vi "Auto Get Server Message and Update UI.vi"(8 "error in (no error)":errorcluster, 10 "MQTT Data":T4, 11 "Data Cluster":T1) -> (0 "error out":errorcluster, 3 "Data Out":T1)   [LabVIEW 2017]
uses:
  controls/Auto UI Data.ctl
  controls/Configuration Details.ctl
  IPC/MQTT/Controls/Publish data.ctl
  <vilib>/vision/Image Controls.llb/IMAQ Image.ctl
  controls/Server CMDs to Publish.ctl
  Database/Controls/DB Options.ctl
panel:
  out "Image Out":T3
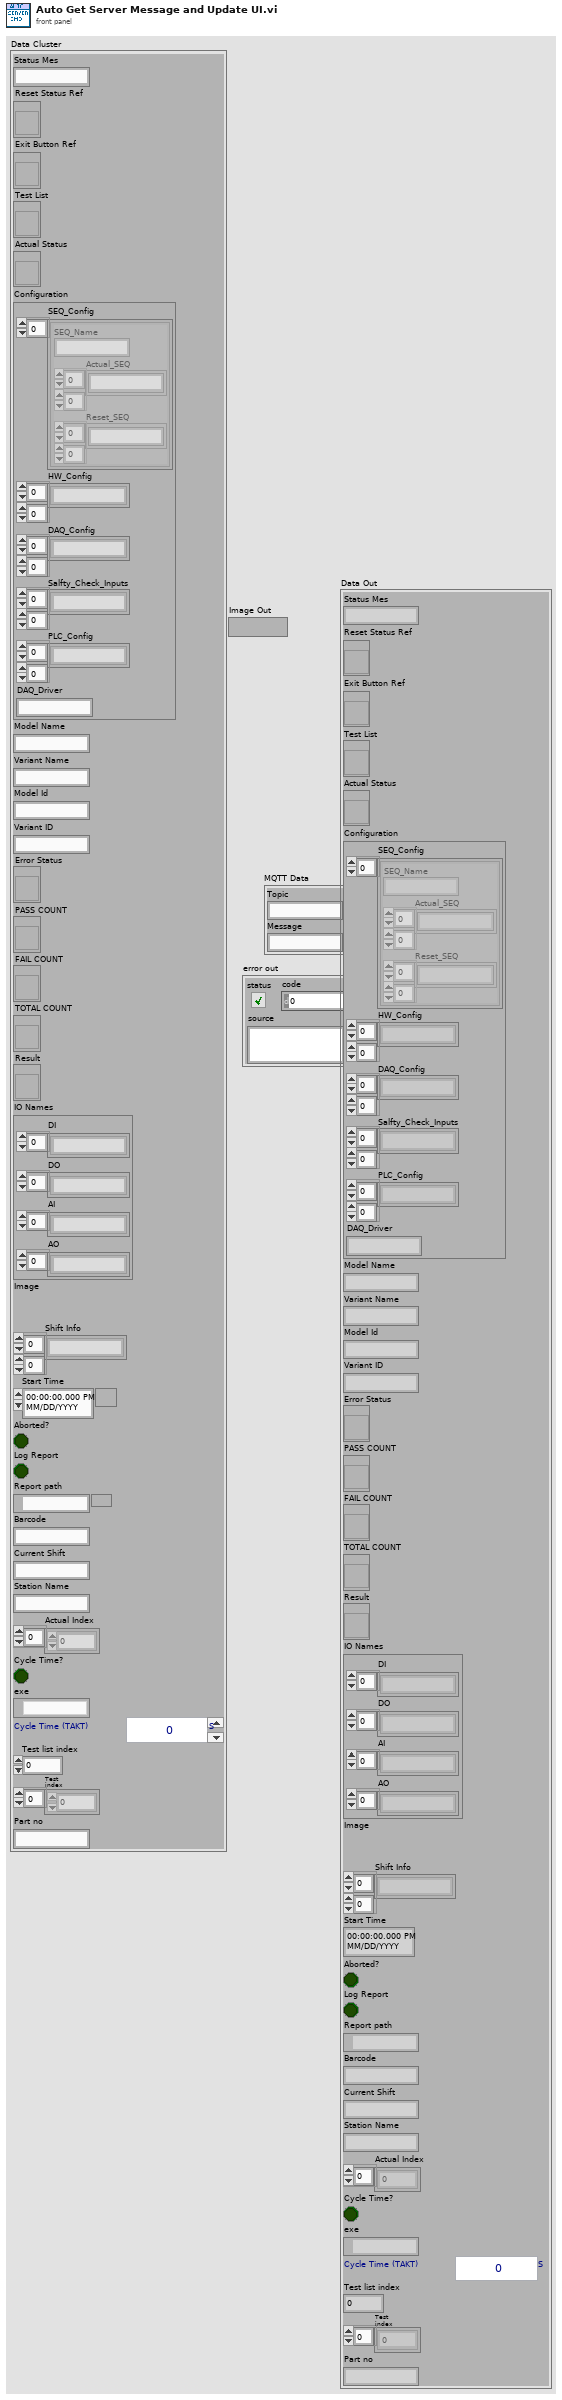
[diagram p1: front panel]
types:
  T1 = typedef "Auto UI Data.ctl" = cluster{"Status Mes":string, "Reset Status Ref":refnum<vi>, "Exit Button Ref":refnum<vi>, "Test List":refnum<vi>, "Actual Status":refnum<vi>, "Configuration":T2, "Model Name":string, "Variant Name":string, "Model Id":string, "Variant ID":string, "Error Status":refnum<vi>, "PASS COUNT":refnum<vi>, "FAIL COUNT":refnum<vi>, "TOTAL COUNT":refnum<vi>, "Result":refnum<vi>, "IO Names":cluster{"DI":string[], "DO":string[], "AI":string[], "AO":string[]}, "Image":T3, "Shift Info":string[][], "Start Time":timestamp, "Aborted?":bool, "Log Report":bool, "Report path":path, "Barcode":string, "Current Shift":string, "Station Name":string, "Actual Index":i32[], "Cycle Time?":bool, "exe":path, "Cycle Time (TAKT)":u16, "Test list index":u32, "Test index":u32[], "Part no":string}
  T2 = typedef "Configuration Details.ctl" = cluster{"SEQ_Config":cluster{"SEQ_Name":string, "Actual_SEQ":string[][], "Reset_SEQ":string[][]}[], "HW_Config":string[][], "DAQ_Config":string[][], "Salfty_Check_Inputs":string[][], "PLC_Config":string[][], "DAQ_Driver":string}
  T3 = typedef "IMAQ Image.ctl" = refnum<image>
  T4 = typedef "Publish data.ctl" = cluster{"Topic":string, "Message":string}
  T5 = cluster{"DI":string[], "DO":string[], "AI":string[], "AO":string[]}
  T6 = cluster{"SEQ_Name":string, "Actual_SEQ":string[][], "Reset_SEQ":string[][]}[]
  T7 = enum8{"Enabled", "Disabled", "Disabled and Grayed Out"}
  T8 = cluster{"Model Name":string, "Variant Name":string}
  T9 = cluster{"Pass/Fail":string, "Cycle time":string, "Model":string, "Variant name":string, "Start time":string, "st":string}
  T10 = typedef "DB Options.ctl" = enum16{"Select", "Execute", "Special Q", "Insert", "Update", "Delete", "Open", "Close"}
  T11 = typedef "Server CMDs to Publish.ctl" = u16
  T12 = typedef "Seq Status to publish.ctl" = cluster{"SEQ Name":string, "Step No":i32, "Step Result":string[][], "Display Message":string, "CMD":T11}
  T13 = typedef "Image Type" = u32
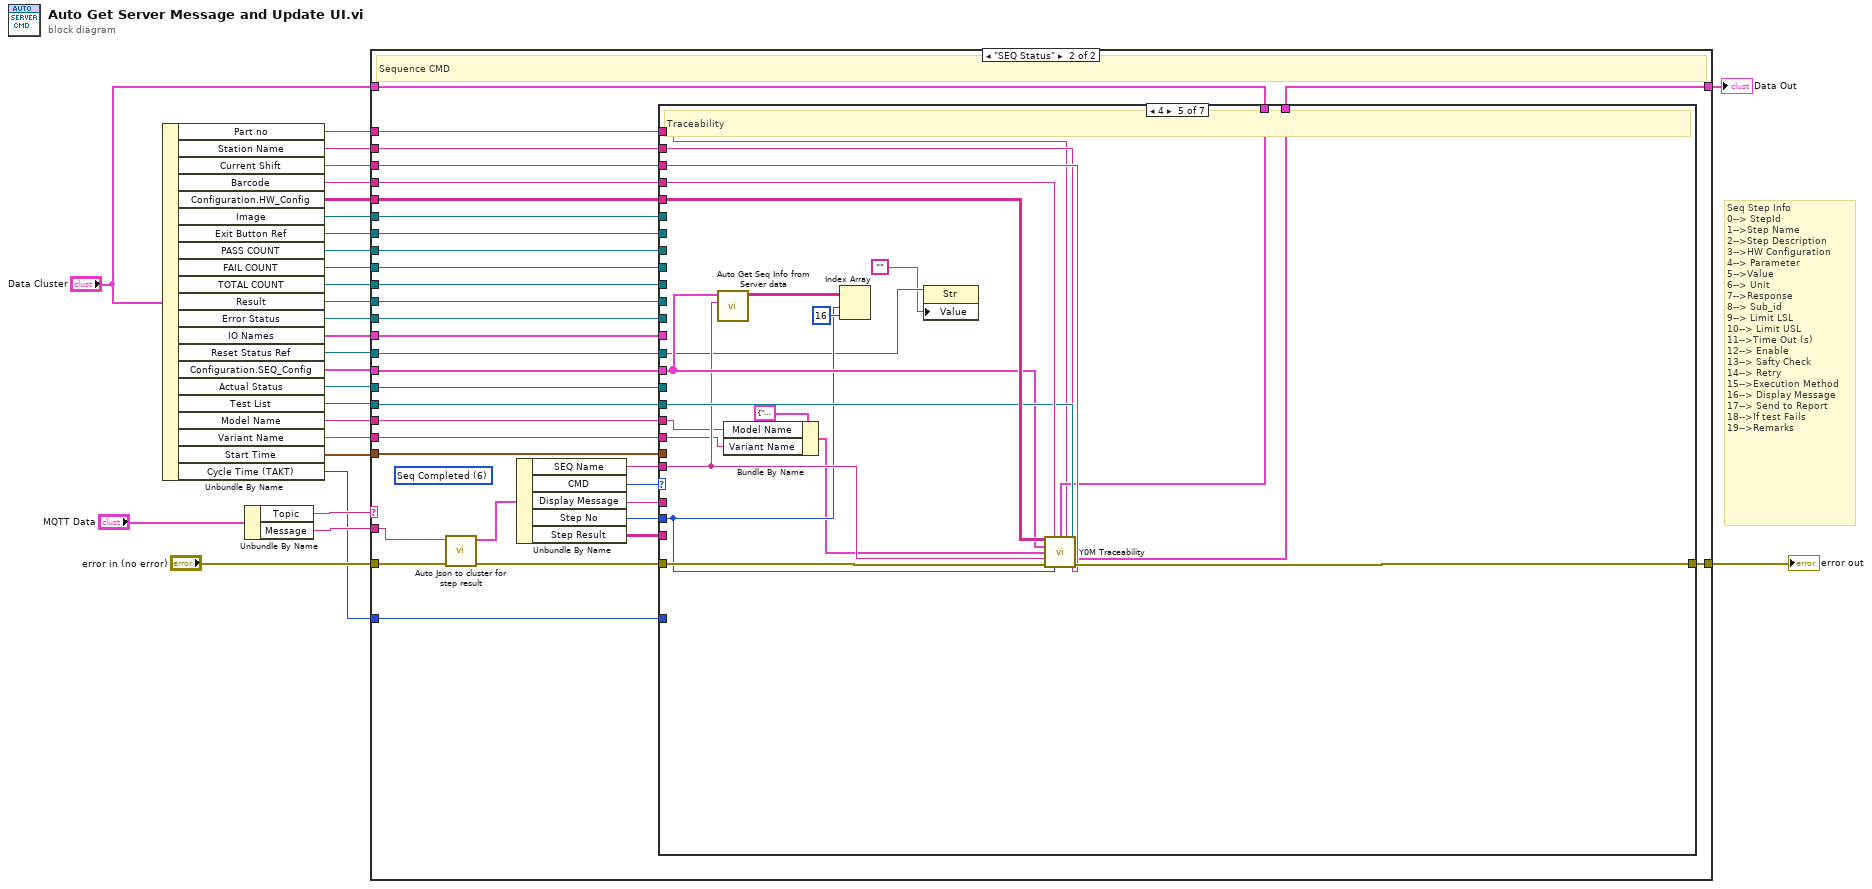
[diagram p0: block diagram]
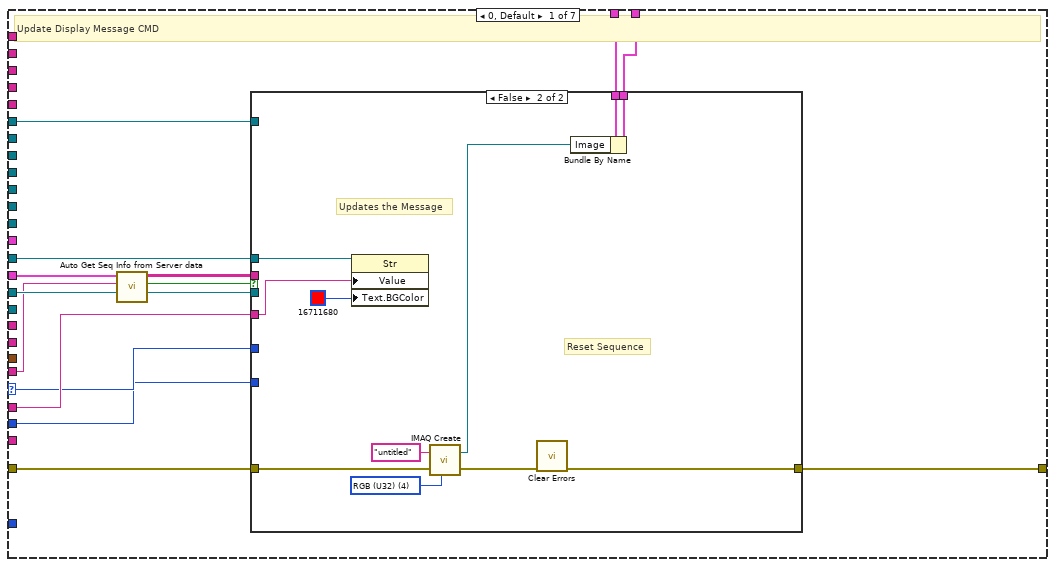
[diagram p3: hidden frame]
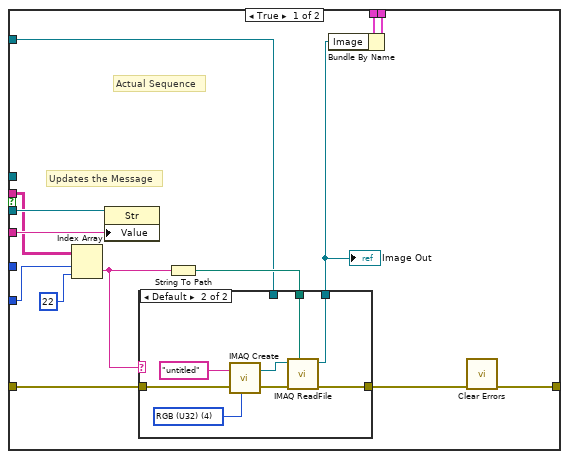
[diagram p4: hidden frame]
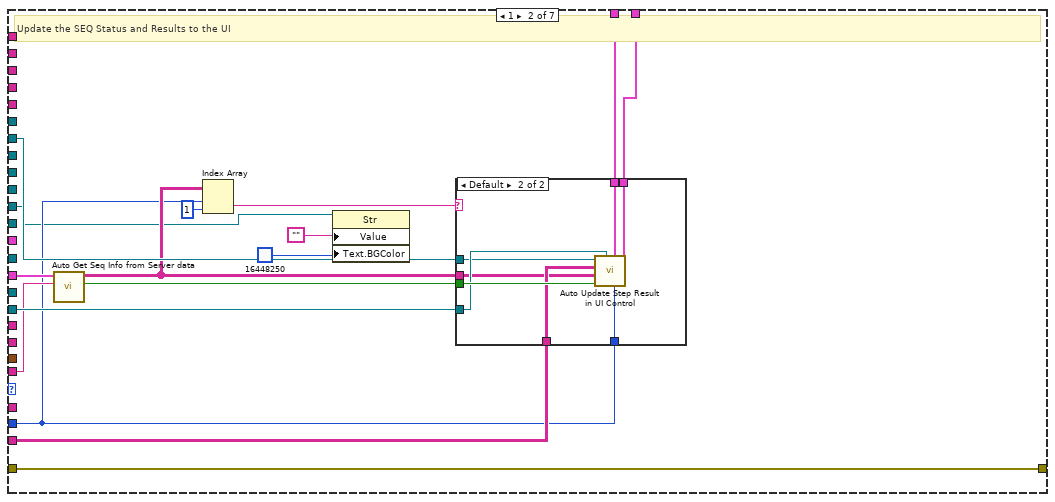
[diagram p6: hidden frame]
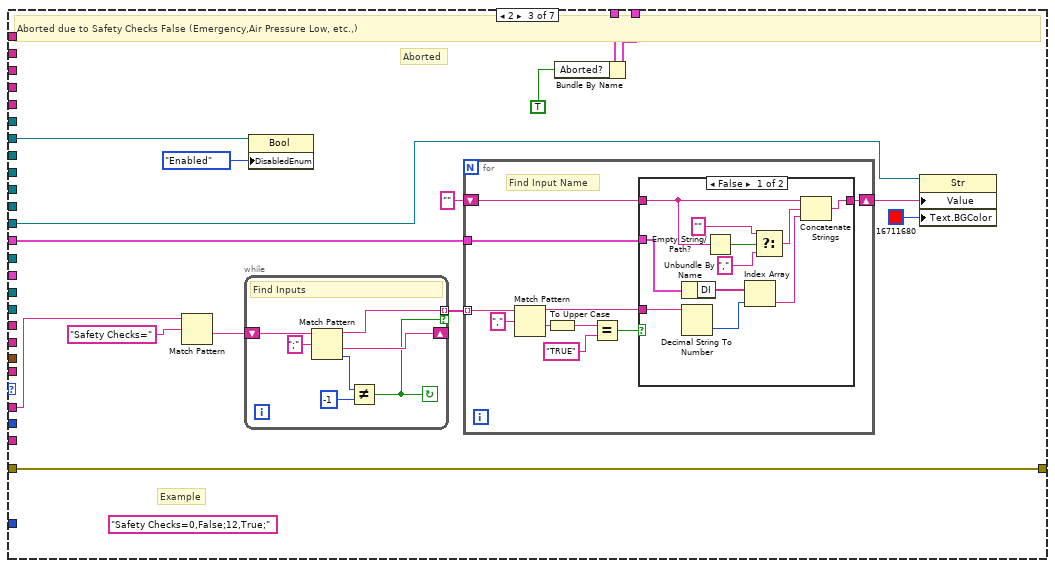
[diagram p8: hidden frame]
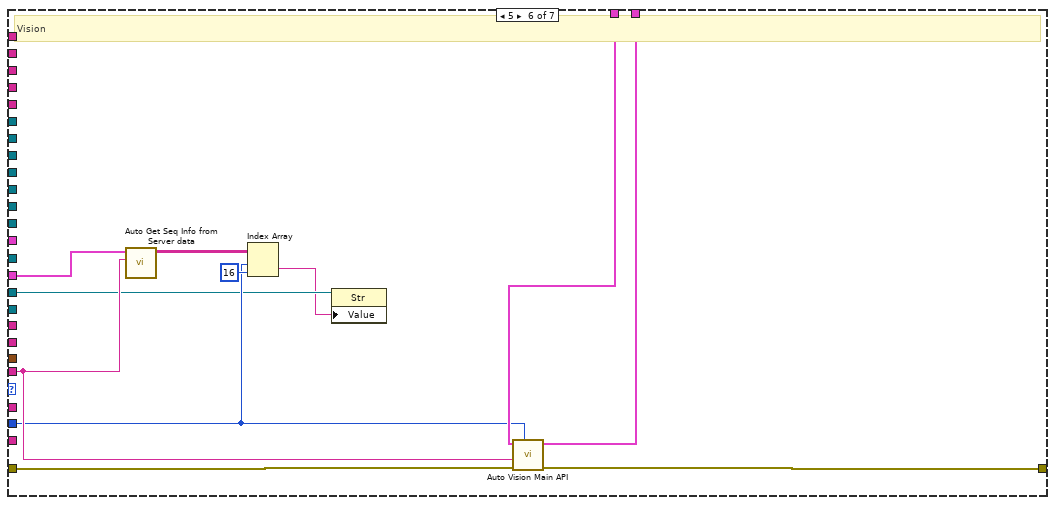
[diagram p11: hidden frame]
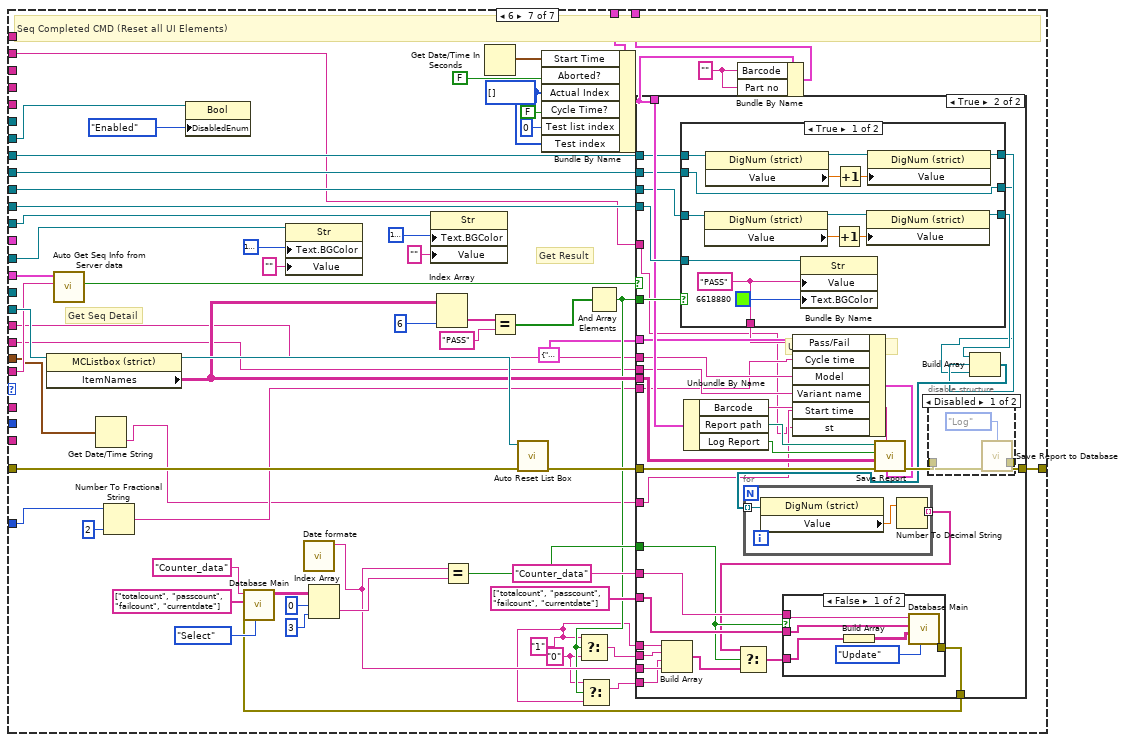
[diagram p12: hidden frame]
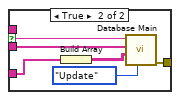
[diagram p15: hidden frame]
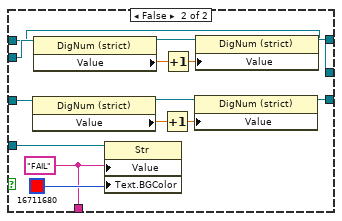
[diagram p16: hidden frame]
diagram:
  # "Seq Step Info\n0--> StepId \n1-->Step Name\t\n2-->Step Description\t\n3-->HW Configuration\n4-->\tParameter\t\n5-->Value\n6-->\tUnit\t\n7-->Response\n8-->\tSub_id\n9-->\tLimit LSL\n10-->\tLimit USL\t\n11-->Time Out (s)\n12-->\tEnable\n13--> Safty Check\n14-->\tRetry\n15-->Execution Method\n16-->\tDisplay Message\n17-->\tSend to Report\t\n18-->If test Fails\n19-->Remarks"
  n1 = Unbundle By Name("Data Cluster") -> ("Part no"=w1:string, "Station Name"=w6:string, "Current Shift"=w7:string, "Barcode"=w8:string, "Configuration.HW_Config"=w9:string[][], "Image"=w12:T3, "Exit Button Ref"=w13:refnum<vi>, "PASS COUNT"=w16:refnum<vi>, "FAIL COUNT"=w15:refnum<vi>, "TOTAL COUNT"=w14:refnum<vi>, "Result"=w17:refnum<vi>, "Error Status"=w18:refnum<vi>, "IO Names"=w19:T5, "Reset Status Ref"=w20:refnum<vi>, "Configuration.SEQ_Config"=w21:T6, "Actual Status"=w28:refnum<vi>, "Test List"=w25:refnum<vi>, "Model Name"=w5:string, "Variant Name"=w4:string, "Start Time"=w3:timestamp, "Cycle Time (TAKT)"=w2:u16)
  n2 = Unbundle By Name("MQTT Data") -> ("Topic"=w23:string, "Message"=w24:string)
  n3 = case shown="\"SEQ Status\"" w23 {
    tunnel: w24 -> [_ w45]
    tunnel: w25 -> [_ w55]
    tunnel: "error in (no error)" -> [w30 w43]
    tunnel: [w30 w60] -> w27
    tunnel: w28 -> [_ w62]
    tunnel: w21 -> [_ w59]
    tunnel: w20 -> [_ w54]
    tunnel: w19 -> [_ w53]
    tunnel: w18 -> [_ w52]
    tunnel: w17 -> [_ w51]
    tunnel: w16 -> [_ w50]
    tunnel: w15 -> [_ w49]
    tunnel: w14 -> [_ w48]
    tunnel: w13 -> [_ w47]
    tunnel: w12 -> [_ w42]
    tunnel: "Data Cluster" -> [w29 w41]
    tunnel: [w29 w40] -> w10
    tunnel: w9 -> [_ w39]
    tunnel: w8 -> [_ w38]
    tunnel: w7 -> [_ w37]
    tunnel: w6 -> [_ w36]
    tunnel: w5 -> [_ w35]
    tunnel: w4 -> [_ w34]
    tunnel: w3 -> [_ w33]
    tunnel: w2 -> [_ w32]
    tunnel: w1 -> [_ w31]
    frame Default {
    }
    frame "SEQ Status" {
      (unwired) T11 6 items=["Display Message", "Step Result", "Aborted", "Log Report", "Traceability", "Vision", "Seq Completed", "Print"] ("CMD")
      # "Sequence CMD"
      n4 = call "Auto Json to cluster for step result.vi"("error in (no error)"=w43, "Message"=w45) -> ("error out"=w46:errorcluster, "SEQ Status"=w44:T12)  [unwired: 8 in]
      n5 = Unbundle By Name(w44) -> ("SEQ Name"=w58:string, "CMD"=w63:T11, "Display Message"=w61:string, "Step No"=w57:i32, "Step Result"=w56:string[][])
      n6 = case shown="4" w63 {
        selector: w63 -> [w69 _ _ _ _ _ _]
        tunnel: w62 -> [w77 _ _ _ _ w206 _]
        tunnel: w61 -> [w76 _ w151 _ _ _ _]
        tunnel: w55 -> [_ w125 _ _ w200 _ w275]
        tunnel: w56 -> [_ w124 _ _ _ _ _]
        tunnel: w46 -> [w68 w128 w152 w183 w204 w215 w256]
        tunnel: [w67 w128 w152 w183 w203 w214 w250] -> w60
        tunnel: w57 -> [w64 w118 _ _ w193 w207 _]
        tunnel: w59 -> [w75 w127 _ _ w195 w211 w267]
        tunnel: w58 -> [w74 w123 _ _ w194 w210 w266]
        tunnel: w54 -> [w72 _ _ _ w192 _ w268]
        tunnel: w53 -> [_ _ w146 _ _ _ _]
        tunnel: w52 -> [_ _ w145 _ _ _ w273]
        tunnel: w51 -> [_ w113 _ _ _ _ w260]
        tunnel: w50 -> [_ _ _ _ _ _ w263]
        tunnel: w49 -> [_ _ _ _ _ _ w262]
        tunnel: w48 -> [_ _ _ _ _ _ w261]
        tunnel: w47 -> [_ w120 w141 _ _ _ w248]
        tunnel: w42 -> [w71 _ _ _ _ _ _]
        tunnel: w41 -> [w66 w122 w140 w182 w187 w213 w252]
        tunnel: [w65 w121 w139 w182 w186 w212 w246] -> w40
        tunnel: w39 -> [_ _ _ _ w202 _ _]
        tunnel: w38 -> [_ _ _ _ w201 _ _]
        tunnel: w37 -> [_ _ _ _ w199 _ _]
        tunnel: w36 -> [_ _ _ _ w198 _ w219]
        tunnel: w35 -> [_ _ _ _ w190 _ w227]
        tunnel: w34 -> [_ _ _ _ w189 _ w226]
        tunnel: w33 -> [_ _ _ _ _ _ w221]
        tunnel: w32 -> [_ _ _ _ _ _ w224]
        tunnel: w31 -> [_ _ _ _ w184 _ _]
        frame 0, Default {
          # "Update Display Message CMD"
          n7 = call "Auto Get Seq Info from Server data.vi"("SEQ Name"=w74, "SEQ_Config"=w75) -> ("Acutal(T)/Reset(F)?"=w73:bool, "Reset_SEQ"=w70:string[][])  [unwired: 8 in]
          n8 = case shown="False" w73 {
            tunnel: w77 -> [w91 _]
            tunnel: w76 -> [w90 w112]
            tunnel: w72 -> [_ w111]
            tunnel: w71 -> [w80 _]
            tunnel: w70 -> [w85 _]
            tunnel: w69 -> [_ _]
            tunnel: w68 -> [w79 w108]
            tunnel: [w86 w103] -> w67
            tunnel: w66 -> [w84 w109]
            tunnel: [w82 w105] -> w65
            tunnel: w64 -> [w81 _]
            frame True {
              # "Actual Sequence"
              # "Updates the Message"
              n9 = Index Array(array=w85, index (row)=w81, index (col)=22 ("disabled index (col)")) -> (element=w78:string)
              n10 = property class="Str"(reference=w91, "Value"=w90) -> ()  [unwired: 1 in, 2 out]
              n11 = String To Path(string=w78) -> (path=w88:path)
              n12 = case shown="Default" w78 {
                tunnel: [w92 w101] -> w89
                tunnel: w88 -> [_ w100]
                tunnel: [w93 w99] -> w83
                tunnel: w80 -> [w93 _]
                tunnel: w79 -> [w92 w98]
                frame "" {
                }
                frame Default {
                  w94 = T13 4 items=["Grayscale (U8)", "Grayscale (I16)", "Grayscale (SGL)", "Complex (CSG)", "RGB (U32)", "HSL (U32)", "RGB (U64)", "Grayscale (U16)"] ("Image Type")
                  n13 = call "IMAQ Create"("Image Name"="untitled", "Image Type"=w94, "error in (no error)"=w98) -> ("New Image"=w95:T3, "error out"=w97:errorcluster)  [unwired: 2 in]
                  n14 = call "IMAQ ReadFile"("File Path"=w100, "error in (no error)"=w97, "Image"=w95) -> ("error out"=w101:errorcluster, "Image Out"=w99:T3)  [unwired: 4 in, 3 out]
                }
              }
              "Image Out" <- w83
              n15 = Bundle By Name(cluster=w84, "Image"=w83) -> (w82:T1)
              n16 = call <vilib>:"Clear Errors.vi"("error in (no error)"=w89) -> ("error out"=w86:errorcluster)  [unwired: 5 in, 1 out]
            }
            frame False {
              w102 = T13 4 items=["Grayscale (U8)", "Grayscale (I16)", "Grayscale (SGL)", "Complex (CSG)", "RGB (U32)", "HSL (U32)", "RGB (U64)", "Grayscale (U16)"] ("Image Type")
              # "Reset Sequence"
              # "Updates the Message"
              n17 = property class="Str"(reference=w111, "Value"=w112, "Text.BGColor"=u32 16711680) -> ()  [unwired: 1 in, 2 out]
              n18 = call "IMAQ Create"("Image Name"="untitled", "Image Type"=w102, "error in (no error)"=w108) -> ("New Image"=w104:T3, "error out"=w107:errorcluster)  [unwired: 2 in]
              n19 = call <vilib>:"Clear Errors.vi"("error in (no error)"=w107) -> ("error out"=w103:errorcluster)  [unwired: 5 in, 1 out]
              n20 = Bundle By Name(cluster=w109, "Image"=w104) -> (w105:T1)
            }
          }
        }
        frame 1 {
          # "Update the SEQ Status and Results to the UI"
          n21 = call "Auto Get Seq Info from Server data.vi"("SEQ Name"=w123, "SEQ_Config"=w127) -> ("Acutal(T)/Reset(F)?"=w126:bool, "Reset_SEQ"=w119:string[][])  [unwired: 8 in]
          n22 = Index Array(array=w119, index (row)=w118, index (col)=1 ("disabled index (col)")) -> (element=w116:string)
          n23 = property class="Str"(reference=w113, "Value"="", "Text.BGColor"=u32 16448250) -> ()  [unwired: 1 in, 2 out]
          n24 = case shown="Default" w116 {
            tunnel: w126 -> [_ w137]
            tunnel: w125 -> [_ w136]
            tunnel: w124 -> [_ w135]
            tunnel: w122 -> [w129 w134]
            tunnel: [w129 w133] -> w121
            tunnel: w120 -> [_ w132]
            tunnel: w119 -> [_ w131]
            tunnel: w118 -> [_ w130]
            frame "Traceability", "Vision" {
            }
            frame Default {
              n25 = call "Auto Update Step Result in UI Control.vi"("Step No"=w130, "Data Cluster in"=w134, "Test List"=w136, "Acutal(T)/Reset(F)?"=w137, "Reset_SEQ"=w131, "Step Result"=w135, "Boolean in"=w132) -> ("Data Cluster out"=w133:T1)  [unwired: 4 in]
            }
          }
        }
        frame 2 {
          (unwired) "Safety Checks=0,False;12,True;"
          # "Aborted"
          # "Example"
          # "Aborted due to Safety Checks False (Emergency,Air Pressure Low, etc.,)"
          n26 = Match Pattern(string=w151, regular expression="Safety Checks=") -> (after substring=w149:string)  [unwired: 1 in, 3 out]
          n27 = while {
            shift-right: [w179] -> _
            shift-left: w149 -> [w181]
            tunnel: [w176] -> w148 mode=indexing if=w175
            stop <- w175 continue-if-true
            # "Find Inputs"
            n28 = Match Pattern(string=w181, regular expression=";") -> (before substring=w176:string, after substring=w179:string, offset past match=w178:i32)  [unwired: 1 in, 1 out]
            n29 = Not Equal?(x=w178, y=-1) -> (x != y?=w175:bool)
          }
          n30 = property class="Bool"(reference=w141, "DisabledEnum"=T7."Enabled" ("Disabled")) -> ()  [unwired: 1 in, 2 out]
          n31 = for {
            tunnel: w148 -> [w162] mode=indexing
            tunnel: w146 -> [w155]
            shift-right: [w153] -> w144
            shift-left: "" ("String") -> [w154]
            # "Find Input Name"
            n32 = Match Pattern(string=w162, regular expression=",") -> (before substring=w156:string, after substring=w160:string)  [unwired: 1 in, 2 out]
            n33 = To Upper Case(1:w160) -> (0:w158:string)
            n34 = Equal?(x=w158, y="TRUE") -> (x = y?=w157:bool)
            n35 = case shown="False" w157 {
              tunnel: w156 -> [w172 _]
              tunnel: w155 -> [w173 _]
              tunnel: w154 -> [w167 w174]
              tunnel: [w169 w174] -> w153
              frame False {
                n36 = Unbundle By Name(w173) -> ("DI"=w171:string[])
                n37 = Decimal String To Number(string=w172) -> (number=w170:i32)  [unwired: 2 in, 1 out]
                n38 = Empty String/Path?(string/path=w167) -> (empty?=w166:bool)
                n39 = Index Array(array=w171, index=w170) -> (element=w168:string)
                n40 = Select(t="" ("string"), s=w166, f="," ("string")) -> (s? t:f=w163:string)
                n41 = Concatenate Strings(w167, w163, w168) -> (w169:string)
              }
              frame True {
              }
            }
          }
          n42 = Bundle By Name(cluster=w140, "Aborted?"=TRUE) -> (w139:T1)
          n43 = property class="Str"(reference=w145, "Value"=w144, "Text.BGColor"=u32 16711680) -> ()  [unwired: 1 in, 2 out]
        }
        frame 3 {
        }
        frame 4 {
          # "Traceability"
          n44 = call "Auto Get Seq Info from Server data.vi"("SEQ Name"=w194, "SEQ_Config"=w195) -> ("Reset_SEQ"=w197:string[][])  [unwired: 8 in, 1 out]
          n45 = Bundle By Name(cluster=T8 {"Model Name"="", "Variant Name"=""} ("Model/Variant"), "Model Name"=w190, "Variant Name"=w189) -> (w188:T8)
          n46 = Index Array(array=w197, index (row)=w193, index (col)=16 ("disabled index (col)")) -> ()  [unwired: 1 out]
          n47 = property class="Str"(reference=w192, "Value"="") -> ()  [unwired: 1 in, 2 out]
          n48 = call "Y0M Traceability.vi"("HW_Config"=w202, "Barcode"=w201, "Data Cluster"=w187, "Part no"=w184, "station_Name"=w198, "SEQ_Config"=w195, "Test List"=w200, "Model/Variant"=w188, "Shift"=w199, "SEQ Name"=w194, "error in (no error)"=w204, "Step No"=w193) -> ("Data Cluster out"=w186:T1, "error out"=w203:errorcluster)  [unwired: 2 in]
        }
        frame 5 {
          # "Vision"
          n49 = call "Auto Get Seq Info from Server data.vi"("SEQ Name"=w210, "SEQ_Config"=w211) -> ("Reset_SEQ"=w209:string[][])  [unwired: 8 in, 1 out]
          n50 = Index Array(array=w209, index (row)=w207, index (col)=16 ("disabled index (col)")) -> (element=w205:string)
          n51 = property class="Str"(reference=w206, "Value"=w205) -> ()  [unwired: 1 in, 2 out]
          n52 = call "Auto Vision Main API.vi"("Step No"=w207, "error in (no error)"=w215, "SEQ Name"=w210, "Data Cluster in"=w213) -> ("error out"=w214:errorcluster, "Data Cluster out"=w212:T1)  [unwired: 6 in]
        }
        frame 6 {
          w230 = "0" ("f")
          w229 = "1"
          w217 = i32[] [] ("Actual Index")
          w216 = "" ("Barcode")
          # "Get Seq Detail"
          # "Get Result"
          # "Seq Completed CMD (Reset all UI Elements)"
          n53 = property class="MCListbox (strict)"(reference=w275) -> (reference out=w274:refnum<vi>, "ItemNames"=w253:string[][])  [unwired: 1 in, 1 out]
          n54 = call "Auto Get Seq Info from Server data.vi"("SEQ Name"=w266, "SEQ_Config"=w267) -> ("Acutal(T)/Reset(F)?"=w265:bool)  [unwired: 8 in, 1 out]
          n55 = Get Date/Time String(seconds (now)=w221) -> (time string=w220:string)  [unwired: 2 in, 1 out]
          n56 = Number To Fractional String(number=w224, precision (6)=i16 2) -> (F-format string=w223:string)  [unwired: 2 in]
          n57 = property class="Bool"(reference=w248, "DisabledEnum"=T7."Enabled" ("Disabled")) -> ()  [unwired: 1 in, 2 out]
          n58 = call "Database Main.vi"("Option"=DB_Options."Select", "Column Name"=string[] ["totalcount", "passcount", "failcount", "currentdate"], "table Name/Query"="Counter_data") -> ("error out"=w236:errorcluster, "Data"=w237:string[][])  [unwired: 6 in, 1 out]
          n59 = property class="Str"(reference=w268, "Text.BGColor"=u32 16777226, "Value"="") -> ()  [unwired: 1 in, 2 out]
          n60 = call "Date formate.vi"() -> ("date string 2"=w233:string)  [unwired: 11 in]
          n61 = Index Array(array=w237, index (row)=0 ("disabled index (row)"), index (col)=3 ("disabled index (col)")) -> (element=w235:string)
          n62 = property class="Str"(reference=w273, "Text.BGColor"=u32 16777226, "Value"="") -> ()  [unwired: 1 in, 2 out]
          n63 = Index Array(array=w253, index (col)=6 ("index")) -> (element=w259:string[])  [unwired: 1 in]
          n64 = Equal?(x=w233, y=w235) -> (x = y?=w234:bool)
          n65 = Get Date/Time In Seconds() -> (seconds since 1Jan1904=w255:timestamp)
          n66 = Equal?(x=w259, y="PASS") -> (x = y?=w264:bool[])
          n67 = call "Auto Reset List Box.vi"("error in (no error)"=w256, "MulticolumnListbox in"=w274) -> ("error out"=w251:errorcluster)  [unwired: 9 in]
          n68 = Bundle By Name(cluster=w252, "Start Time"=w255, "Aborted?"=FALSE, "Actual Index"=w217, "Cycle Time?"=FALSE, "Test list index"=u32 0, "Test index"=w217) -> (w249:T1)
          n69 = And Array Elements(Boolean array=w264) -> (logical AND=w231:bool)
          n70 = Select(t=w229, s=w231, f=w230) -> (s? t:f=w232:string)
          n71 = Select(t=w230, s=w231, f=w229) -> (s? t:f=w228:string)
          n72 = case shown="True" w265 {
            tunnel: w231 -> [_ w312]
            tunnel: w263 -> [_ w300]
            tunnel: w262 -> [_ w299]
            tunnel: w261 -> [_ w301]
            tunnel: w260 -> [_ w311]
            tunnel: w253 -> [_ w307]
            tunnel: w249 -> [_ w310]
            tunnel: w251 -> [w276 w308]
            tunnel: [w276 w304] -> w250
            tunnel: "Counter_data" ("table Name/Query") -> [_ w298]
            tunnel: string[] ["totalcount", "passcount", "failcount", "currentdate"] ("Column Name") -> [_ w297]
            tunnel: w236 -> [_ w296]
            tunnel: w234 -> [_ w295]
            tunnel: w233 -> [_ w293]
            tunnel: w229 -> [_ w292]
            tunnel: w232 -> [_ w289]
            tunnel: w228 -> [_ w288]
            tunnel: T9 {"Pass/Fail"="PASS", "Cycle time"="67.86 s", "Model"="Y1k s", "Variant name"="Y1k_LO-MT-RHS-CNG-0N39", "Start time"="Y1k_LO-MT-RHS-CNG-0N39", "st"=""} ("In cluster 2") -> [_ w287]
            tunnel: w227 -> [_ w285]
            tunnel: w226 -> [_ w284]
            tunnel: w220 -> [_ w282]
            tunnel: w223 -> [_ w281]
            tunnel: w219 -> [_ w277]
            frame False {
            }
            frame True {
              # "Update PASS or FAIL"
              n73 = Build Array(w292, w289, w288, w293) -> (w291:string[])
              n74 = case shown="True" w312 {
                tunnel: w300 -> [w343 w345]
                tunnel: w301 -> [w338 w353]
                tunnel: w299 -> [w330 w352]
                tunnel: w311 -> [w335 w349]
                tunnel: [w333 w347] -> w286
                tunnel: [w332 w345] -> w280
                tunnel: [w331 w344] -> w279
                tunnel: [w330 w346] -> w278
                frame True {
                  w333 = "PASS" ("Value")
                  n75 = property class="DigNum (strict)"(reference=w338) -> (reference out=w336:refnum<vi>, "Value"=w339:dbl)  [unwired: 1 in, 1 out]
                  n76 = property class="DigNum (strict)"(reference=w343) -> (reference out=w337:refnum<vi>, "Value"=w342:dbl)  [unwired: 1 in, 1 out]
                  n77 = property class="Str"(reference=w335, "Value"=w333, "Text.BGColor"=u32 6618880) -> ()  [unwired: 1 in, 2 out]
                  n78 = Increment(x=w339) -> (x+1=w340:dbl)
                  n79 = Increment(x=w342) -> (x+1=w341:dbl)
                  n80 = property class="DigNum (strict)"(reference=w336, "Value"=w340) -> (reference out=w331:refnum<vi>)  [unwired: 1 in, 1 out]
                  n81 = property class="DigNum (strict)"(reference=w337, "Value"=w341) -> (reference out=w332:refnum<vi>)  [unwired: 1 in, 1 out]
                }
                frame False {
                  w347 = "FAIL" ("Value")
                  n82 = property class="DigNum (strict)"(reference=w353) -> (reference out=w351:refnum<vi>, "Value"=w354:dbl)  [unwired: 1 in, 1 out]
                  n83 = property class="DigNum (strict)"(reference=w352) -> (reference out=w350:refnum<vi>, "Value"=w357:dbl)  [unwired: 1 in, 1 out]
                  n84 = property class="Str"(reference=w349, "Value"=w347, "Text.BGColor"=u32 16711680) -> ()  [unwired: 1 in, 2 out]
                  n85 = Increment(x=w354) -> (x+1=w355:dbl)
                  n86 = Increment(x=w357) -> (x+1=w356:dbl)
                  n87 = property class="DigNum (strict)"(reference=w351, "Value"=w355) -> (reference out=w344:refnum<vi>)  [unwired: 1 in, 1 out]
                  n88 = property class="DigNum (strict)"(reference=w350, "Value"=w356) -> (reference out=w346:refnum<vi>)  [unwired: 1 in, 1 out]
                }
              }
              n89 = Unbundle By Name(w310) -> ("Barcode"=w305:string, "Report path"=w309:path, "Log Report"=w306:bool)
              n90 = Bundle By Name(cluster=w287, "Pass/Fail"=w286, "Cycle time"=w281, "Model"=w285, "Variant name"=w284, "Start time"=w282, "st"=w277) -> (w283:T9)
              n91 = call "Save Report.vi"("In cluster"=w283, "Barcode"=w305, "error in (no error)"=w308, "ItemNames"=w307, "Log Report"=w306, "Report path"=w309) -> ("error out"=w303:errorcluster)  [unwired: 5 in]
              n92 = disable-structure shown="Disabled" {
                disable-tunnel: [w315 _] -> w304
                disable-tunnel: w303 -> [w313 _]
                frame Disabled {
                  n93 = call "Save Report to Database.vi"("Option"=enum16{"Write", "Log", "Log Barcode"}."Log", "error in (no error)"=w313) -> ("error out"=w315:errorcluster)  [unwired: 13 in]
                }
                frame Enabled {
                }
              }
              n94 = Build Array(w279, w280, w278) -> (w302:refnum<vi>[])
              n95 = for {
                tunnel: w302 -> [w329] mode=indexing
                tunnel: [w327] -> w294 mode=indexing
                n96 = property class="DigNum (strict)"(reference=w329) -> ("Value"=w328:dbl)  [unwired: 1 in, 2 out]
                n97 = Number To Decimal String(number=w328) -> (decimal integer string=w327:string)  [unwired: 1 in]
              }
              n98 = Select(t=w294, s=w295, f=w291) -> (s? t:f=w290:string[])
              n99 = case shown="False" w295 {
                tunnel: w298 -> [w317 w326]
                tunnel: w297 -> [w316 w325]
                tunnel: w296 -> [_ w324]
                tunnel: w290 -> [w318 w322]
                frame False {
                  n100 = Build Array(w318) -> (w320:string[][])
                  n101 = call "Database Main.vi"("Option"=DB_Options."Update", "Column Values"=w320, "Column Name"=w316, "table Name/Query"=w317) -> ()  [unwired: 5 in, 3 out]
                }
                frame True {
                  n102 = Build Array(w322) -> (w321:string[][])
                  n103 = call "Database Main.vi"("Option"=DB_Options."Update", "error in (no error)"=w324, "Column Values"=w321, "Column Name"=w325, "table Name/Query"=w326) -> ()  [unwired: 4 in, 3 out]
                }
              }
            }
          }
          n104 = Bundle By Name(cluster=w249, "Barcode"=w216, "Part no"=w216) -> (w246:T1)
        }
      }
    }
  }
  "error out" <- w27
  "Data Out" <- w10
